vi "FuncImg-Export single ROI data.vi"(7 "ROI number":i32, 8 "Error in":errorcluster, 9 "Single ROI data files reorderedin ascending file-name order":path[](array[path]), 11 "Exported tdms file":refnum<k34>) -> (0 "Error out":errorcluster, 2 "Number of data points in single POI (all trials)":i32, 3 "Exported tdms file":refnum<k34>)   [LabVIEW 2017]
uses:
  <userlib>/My Palettes.lib/Files & paths/Spreadsheet/Read From Spreadsheet File (I64)-Mod.vi
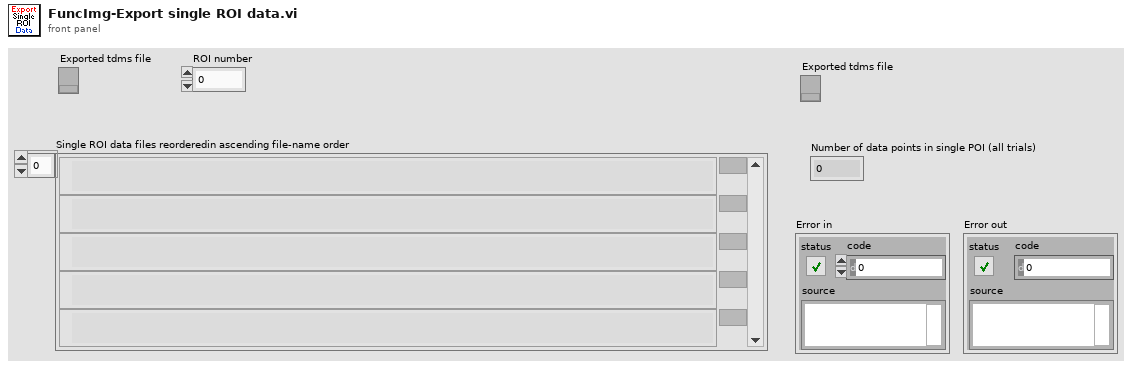
[diagram p1: front panel]
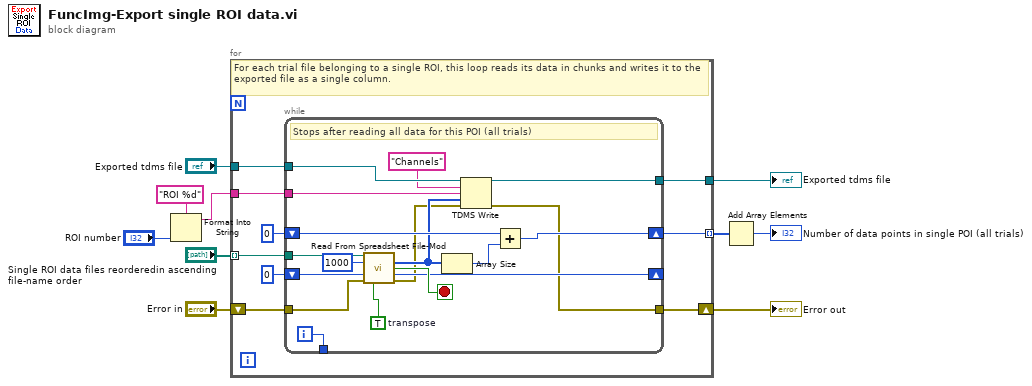
[diagram p0: block diagram]
diagram:
  n1 = Format Into String(format string="ROI %d", "ROI number") -> (resulting string=w3:string)  [unwired: 2 in, 1 out]
  n2 = for {
    tunnel: "Single ROI data files reorderedin ascending file-name order" -> [w19] mode=indexing
    tunnel: [w18] -> w9 mode=indexing
    shift-right: [w15] -> w7
    shift-left: "Error in" -> [w14]
    tunnel: "Exported tdms file" -> [w13]
    tunnel: w3 -> [w12]
    tunnel: [w11] -> w2
    # "For each trial file belonging to a single ROI, this loop reads its data in chunks and writes it to the exported file as a single column."
    n3 = while {
      tunnel: w19 -> [w36]
      shift-right: [w30] -> w18
      shift-left: 0 ("start of read offset (chars.:0)") -> [w33]
      shift-right: [w29] -> _
      shift-left: 0 ("start of read offset (chars.:0)") -> [w35]
      tunnel: [w28] -> _
      tunnel: w14 -> [w27]
      tunnel: [w22] -> w15
      tunnel: w13 -> [w26]
      tunnel: w12 -> [w24]
      tunnel: [w21] -> w11
      i -> [w28]
      stop <- w31 stop-if-true
      w37 = TRUE  # transpose
      # "Stops after reading all data for this POI (all trials)"
      n4 = call-poly <userlib>:"Read From Spreadsheet File-Mod.vi"("file path (dialog if empty)"=w36, "number of rows (all:-1)"=1000, "start of read offset (chars.:0)"=w35, "error in"=w27, "transpose (no:F)"=w37) -> ("first row"=w25:i64[], "EOF?"=w31:bool, "mark after read (chars.)"=w29:i32, "error out"=w23:errorcluster)  [unwired: 5 in, 2 out]
      n5 = Array Size(array=w25) -> (size(s)=w34:i32)
      n6 = TDMS Write(0:w26, 5:"Channels" ("group name"), 7:w24, 9:w25, 11:w23) -> (4:w21:refnum<k34>, 15:w22:errorcluster)  [unwired: 1 in, 2 out]
      n7 = Add(x=w33, y=w34) -> (x+y=w30:i32)
    }
  }
  "Error out" <- w7
  "Exported tdms file" <- w2
  n8 = Add Array Elements(numeric array=w9) -> (sum=→"Number of data points in single POI (all trials)":i32)
